vi "Untitled 1.vi"() -> ()   [LabVIEW 2017]
uses:
  <vilib>/DAQmx/create/channels.llb/DAQmx Create Channel (AI-Voltage-Basic).vi
  <vilib>/DAQmx/configure/timing.llb/DAQmx Timing (Sample Clock).vi
  <vilib>/DAQmx/configure/trigger.llb/DAQmx Start Trigger (Digital Edge).vi
  <vilib>/DAQmx/read.llb/DAQmx Read (Analog 1D Wfm NChan NSamp).vi
  <vilib>/Analysis/NI_AALPro.lvlib
  <vilib>/Analysis/2dsp.llb/Power Spectrum (DBL).vi
panel:
  out "Waveform Chart 3":dbl[](graph)
  in  "Target Path":path=path "C:/Users/klt8/Documents" caption="Final saved file location"
  out "Waveform Chart 2":dbl[](graph)
  out "Waveform Chart":waveform(dbl)[](graph)
  in  "Notes":cluster{"Experimenter":string}
  in  "path":path
  in  "Time (sec)":dbl(knob)=15.0 min=0.0 max=60.0 step=1.0 scale=0.0..60.0 scale format="%#_2g"
  out "Analog Samples":i32
  in  "Analog Acquisition":cluster{"Sampling Rate":u32}={"Sampling Rate"=20000} {"Sampling Rate" format="%0.0f"}
  in  "Channel (AI)":tag="Dev1/ai0:7"
  in  "Analog Channels":string[](array[string])=["Neural_LH", "Force_Sensor", "LPadSol", "RPadSol", "AudSol", "Respiration", "EMG", "Neural_RH"]
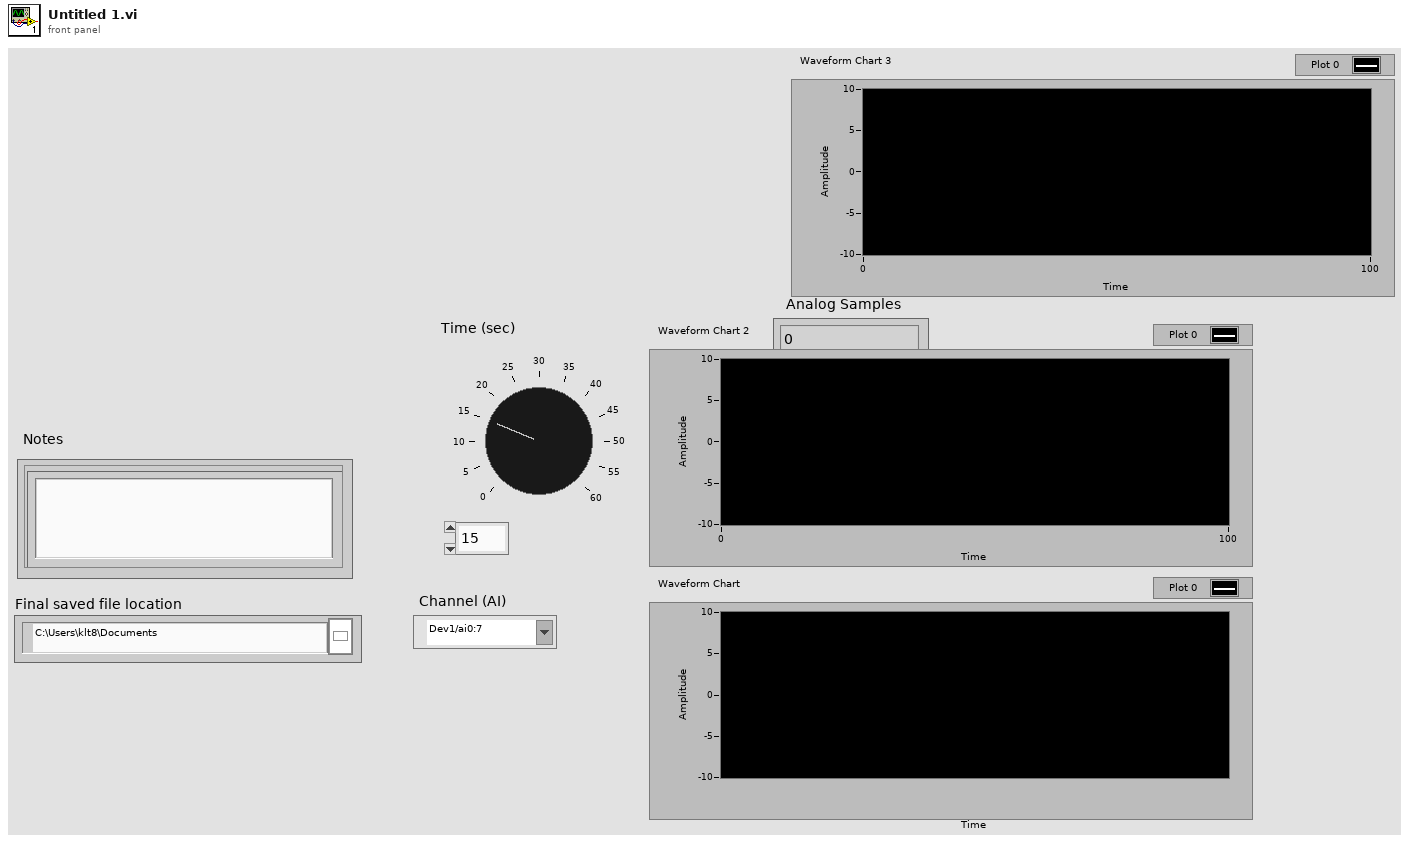
[diagram p1: front panel]
types:
  T1 = enum16{"open", "open or create", "create or replace", "create", "open (read-only)"}
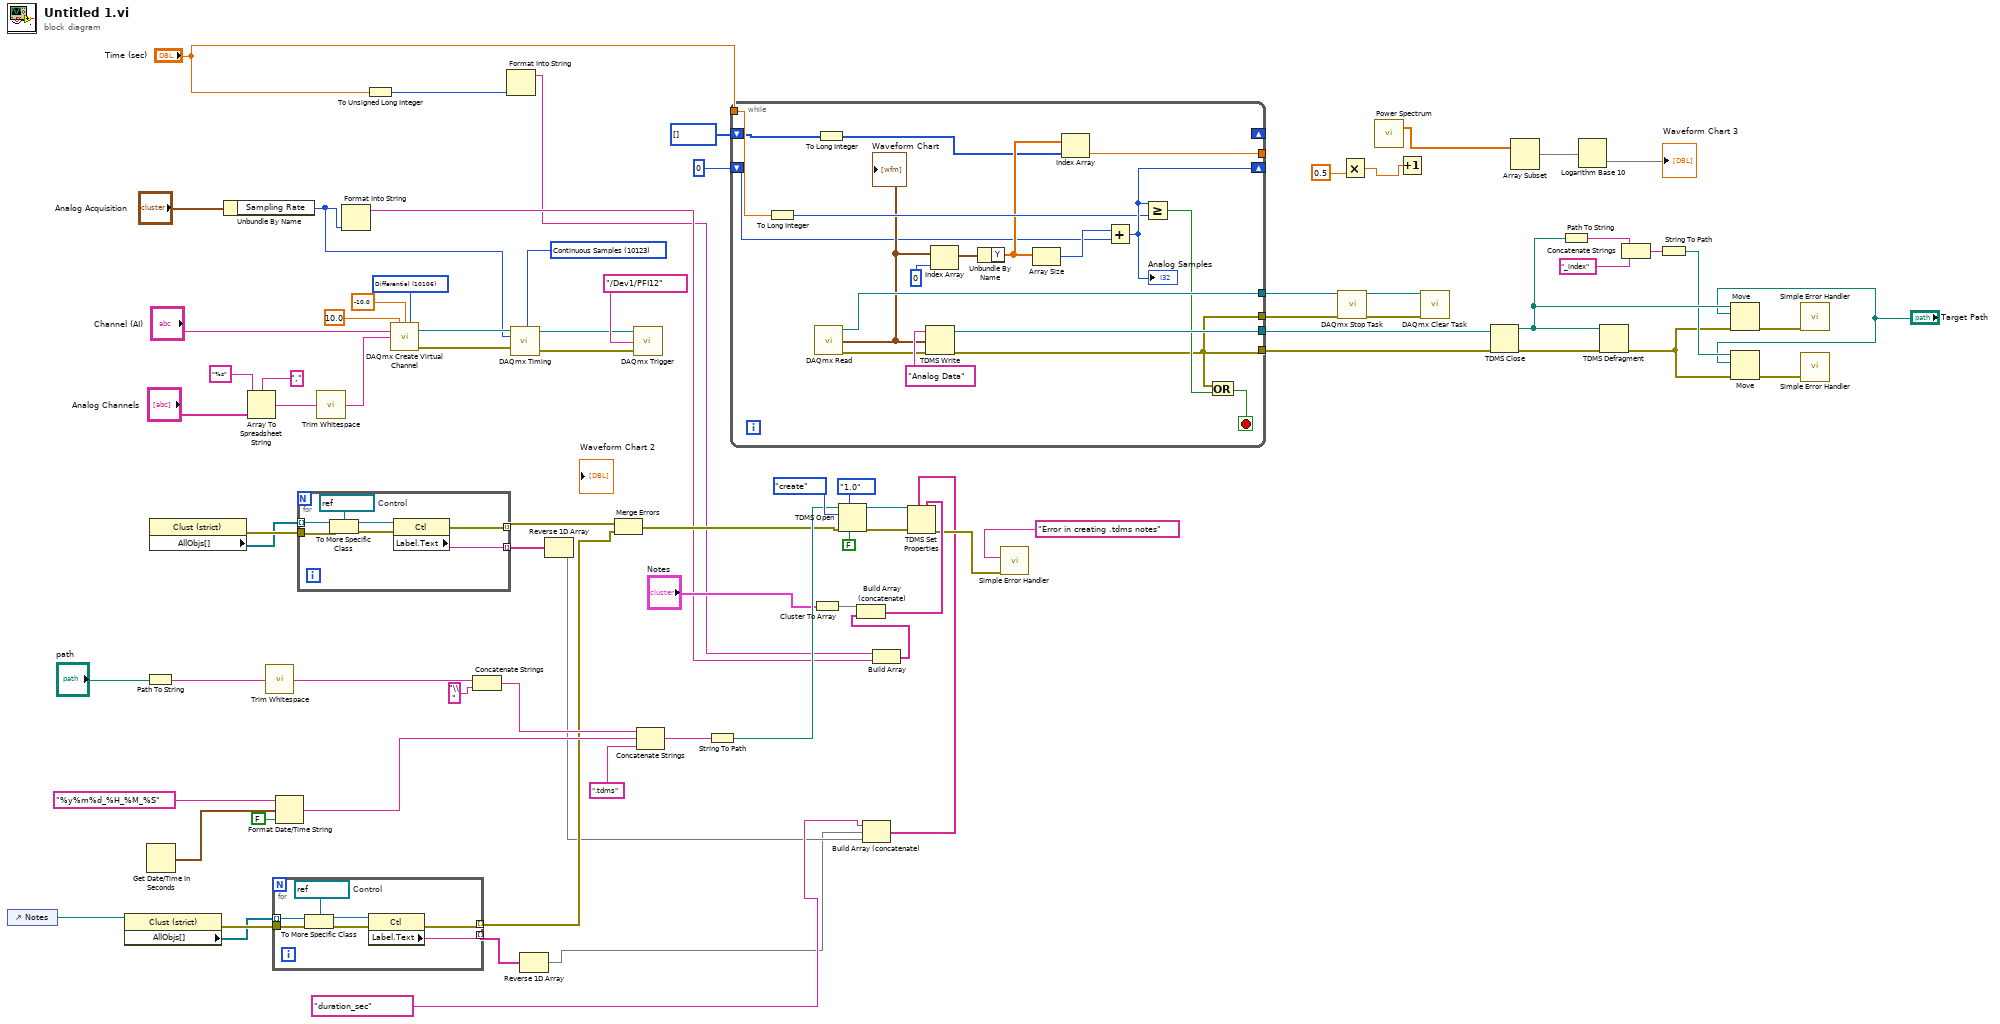
[diagram p0: block diagram]
diagram:
  w78 = 10123 items=["Finite Samples"=10178, "Continuous Samples"=10123, "Hardware Timed Single Point"=12522] ("sample mode")
  w81 = 10106 items=["default"=-1, "RSE"=10083, "NRSE"=10078, "Differential"=10106, "Pseudodifferential"=12529] ("input terminal configuration")
  n1 = control-ref of="Notes"() -> (w31:refnum<vi>)
  n2 = property class="Clust (strict)"(reference=w31) -> (error out=w32:errorcluster, "AllObjs[]"=w30:refnum<vi>[])  [unwired: 1 in, 1 out]
  n3 = Path To String(path="path") -> (string=w42:string)
  n4 = Get Date/Time In Seconds() -> (seconds since 1Jan1904=w46:timestamp)
  n5 = property class="Clust (strict)"() -> (error out=w65:errorcluster, "AllObjs[]"=w63:refnum<vi>[])  [unwired: 2 in, 1 out]
  n6 = Unbundle By Name("Analog Acquisition") -> ("Sampling Rate"=w35:u32)
  n7 = Array To Spreadsheet String(delimiter (Tab)=",", array="Analog Channels", 3:"%s" ("format string")) -> (spreadsheet string=w70:string)
  n8 = call <vilib>:"Trim Whitespace.vi"("string"=w42) -> ("trimmed string"=w40:string)  [unwired: 1 in]
  n9 = for {
    tunnel: [w86] -> w29 mode=indexing
    tunnel: w32 -> [w85]
    tunnel: [w83] -> w26 mode=indexing
    tunnel: w30 -> [w82] mode=indexing
    w87 = refnum<vi> refnum  # Control
    n10 = To More Specific Class(target class=w87, reference=w82, error in=w85) -> (specific class reference=w88:refnum<vi>, error out=w84:errorcluster)
    n11 = property class="Ctl"(reference=w88, error in=w84) -> (error out=w83:errorcluster, "Label.Text"=w86:string)  [unwired: 1 out]
  }
  n12 = Format Date/Time String(time format string (%c)="%y%m%d_%H_%M_%S", seconds (now)=w46, UTC format=FALSE) -> (date/time string=w38:string)
  n13 = for {
    tunnel: [w93] -> w64 mode=indexing
    tunnel: w65 -> [w92]
    tunnel: [w90] -> w33 mode=indexing
    tunnel: w63 -> [w89] mode=indexing
    w94 = refnum<vi> refnum  # Control
    n14 = To More Specific Class(target class=w94, reference=w89, error in=w92) -> (specific class reference=w95:refnum<vi>, error out=w91:errorcluster)
    n15 = property class="Ctl"(reference=w95, error in=w91) -> (error out=w90:errorcluster, "Label.Text"=w93:string)  [unwired: 1 out]
  }
  n16 = call <vilib>:"Trim Whitespace.vi"("string"=w70) -> ("trimmed string"=w69:string)  [unwired: 1 in]
  n17 = Format Into String(w35) -> (resulting string=w24:string)  [unwired: 3 in, 1 out]
  n18 = To Unsigned Long Integer(number="Time (sec)") -> (unsigned 32bit integer=w48:u32)
  n19 = call-poly <vilib>:"DAQmx Create Virtual Channel.vi"("maximum value"=10.0, "minimum value"=-10.0, "input terminal configuration"=w81, "physical channels"="Channel (AI)", "name to assign"=w69) -> ("task out"=w80:refnum<k21>, "error out"=w79:errorcluster)  [unwired: 9 in]
  n20 = Concatenate Strings(w40, "\\" ("string")) -> (w37:string)
  n21 = Format Into String(w48) -> (resulting string=w23:string)  [unwired: 3 in, 1 out]
  n22 = call-poly <vilib>:"DAQmx Timing.vi"("task/channels in"=w80, "sample mode"=w78, "rate"=w35, "error in"=w79) -> ("task out"=w67:refnum<k21>, "error out"=w77:errorcluster)  [unwired: 10 in]
  n23 = Reverse 1D Array(array=w29) -> (reversed array=w20:string[])
  n24 = Reverse 1D Array(array=w64) -> (reversed array=w21:string[])
  n25 = Merge Errors(w33, w26) -> (w27:errorcluster)
  n26 = call-poly <vilib>:"DAQmx Trigger.vi"("task/channels in"=w67, "source"=tag "/Dev1/PFI12", "error in"=w77) -> ()  [unwired: 11 in, 2 out]
  n27 = Concatenate Strings(w37, w38, ".tdms" ("string")) -> (w43:string)
  n28 = String To Path(string=w43) -> (path=w36:path)
  n29 = while {
    tunnel: [w114] -> w7
    tunnel: [w105] -> w8
    tunnel: [w113] -> w53
    shift-right: [w109] -> _
    shift-left: 0 -> [w99]
    tunnel: [w105] -> w50
    tunnel: "Time (sec)" -> [w103]
    shift-right: _ -> [_]
    shift-left: i32[] [] -> [w97]
    tunnel: [w98] -> _
    stop <- w106 stop-if-true
    n30 = To Long Integer(number=w103) -> (32bit integer=w104:i32)
    n31 = call-poly <vilib>:"DAQmx Read.vi"() -> ("task out"=w113:refnum<k21>, "data"=w102:waveform(dbl)[], "error out"=w108:errorcluster)  [unwired: 13 in]
    "Waveform Chart" <- w102
    n32 = To Long Integer(number=w97) -> (32bit integer=w96:i32[])
    n33 = TDMS Write(5:"Analog Data" ("group name in (Untitled)"), 9:w102, 11:w108) -> (4:w114:refnum<k34>, 15:w105:errorcluster)  [unwired: 3 in, 2 out]
    n34 = Index Array(array=w102, index=0) -> (element=w101:waveform(dbl))
    n35 = Unbundle By Name(w101) -> ("Y"=w100:dbl[])
    n36 = Array Size(array=w100) -> (size(s)=w110:i32)
    n37 = Index Array(array=w100, index=w96) -> (element=w98:dbl)
    n38 = Add(x=w110, y=w99) -> (x+y=w109:i32)
    "Analog Samples" <- w109
    n39 = Greater Or Equal?(x=w109, y=w104) -> (x >= y?=w107:bool)
    n40 = Compound Arithmetic op=OR(w105, w107) -> (w106:bool)
  }
  n41 = Cluster To Array(cluster="Notes") -> (array=w62:string[])
  n42 = TDMS Open(6:FALSE ("disable buffering? (T)"), 7:enum16{"1.0", "2.0"}."1.0" ("file format version (2.0)"), 8:w27, 10:T1."create" ("operation (0:open)"), 11:w36) -> (0:w57:errorcluster, 3:w58:refnum<k34>)  [unwired: 2 in]
  n43 = Build Array (concatenate)("duration_sec", w20, w21) -> (w19:string[])
  n44 = Build Array(w23, w24) -> (w25:string[])
  n45 = Build Array (concatenate)(w62, w25) -> (w56:string[])
  n46 = TDMS Set Properties(5:w56, 7:w19, 8:w57, 11:w58) -> (0:w55:errorcluster)  [unwired: 2 in, 3 out]
  n47 = call <vilib>:"Simple Error Handler.vi"("error source (\" \")"="Error in creating .tdms notes" ("error source (\" \")"), "error in (no error)"=w55) -> ()  [unwired: 3 in, 5 out]
  n48 = call <vilib>:"DAQmx Stop Task.vi"("task/channels in"=w53, "error in"=w50) -> ("task out"=w52:refnum<k21>, "error out"=w51:errorcluster)  [unwired: 12 in]
  n49 = Multiply(y=0.5) -> (x*y=w4:dbl)  [unwired: 1 in]
  n50 = call-poly <vilib>:"Power Spectrum.vi"() -> ("Power Spectrum"=w6:dbl[])  [unwired: 1 in, 1 out]
  n51 = Increment(x=w4) -> ()  [unwired: 1 out]
  n52 = call <vilib>:"DAQmx Clear Task.vi"("task in"=w52, "error in"=w51) -> ()  [unwired: 13 in, 1 out]
  n53 = TDMS Close(8:w8, 11:w7) -> (0:w18:errorcluster, 3:w14:path)
  n54 = Array Subset(array=w6) -> (w5:dbl[])  [unwired: 2 in]
  n55 = Path To String(path=w14) -> (string=w16:string)
  n56 = Logarithm Base 10(1:w5) -> (0:→"Waveform Chart 3":dbl[])
  n57 = TDMS Defragment(4:w18, 7:w14) -> (0:w11:errorcluster)
  n58 = Concatenate Strings(w16, "_index" ("string")) -> (w13:string)
  n59 = String To Path(string=w13) -> (path=w12:path)
  n60 = Move(source path=w14, error in=w11, 10:"Target Path") -> (error out=w17:errorcluster)  [unwired: 2 in, 2 out]
  n61 = Move(source path=w12, error in=w11, 10:"Target Path") -> (error out=w10:errorcluster)  [unwired: 2 in, 2 out]
  n62 = call <vilib>:"Simple Error Handler.vi"("error in (no error)"=w17) -> ()  [unwired: 1 in, 8 out]
  n63 = call <vilib>:"Simple Error Handler.vi"("error in (no error)"=w10) -> ()  [unwired: 1 in, 8 out]
